vi "test_SessionInitializeErrors_CallCreateSessions_CloseCalledForPreviouslyInitializedSessionsWithProperBehavior.vi"(8 "error in":errorcluster) -> (0 "error out":errorcluster, 2 "result":string, 3 "pass":bool)   [LabVIEW 2020, in "MeasurementServerTests.lvlib"]
uses:
  MeasurementServerTests.lvlib
  da6ffb6f-c1c9-4957-84dd-e9228483c454.vi
  ffc64c76-1568-41a3-8328-b9126ac9a28d.vi
  Helpers/Fake Instrument/Fake Instrument.lvclass
  \\tsclient\C/dev/measurementlink-labview/Source/Runtime/MeasurementLink Instrument/IInstrument/IInstrument.lvclass
  Runtime/MeasurementLink Session Management/Session Reservation/Create Sessions Impl.vi
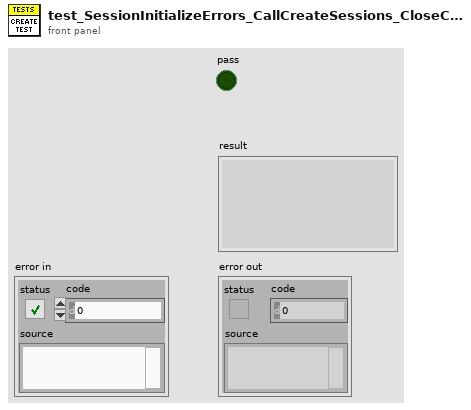
[diagram p1: front panel]
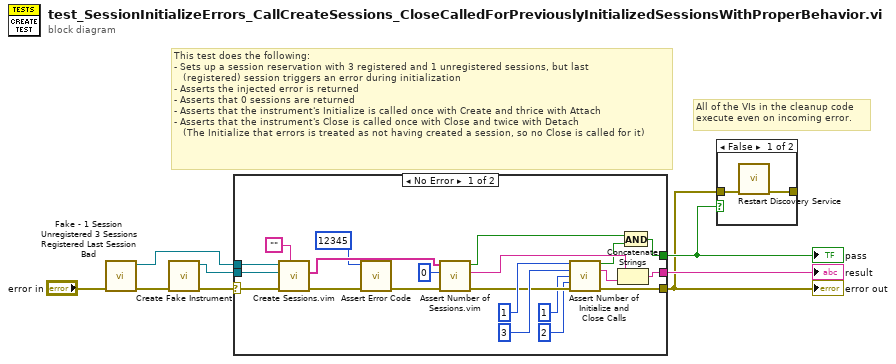
[diagram p0: block diagram]
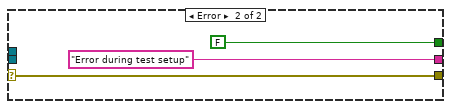
[diagram p2: hidden frame]
diagram:
  # "All of the VIs in the cleanup code\nexecute even on incoming error."
  # "This test does the following:\n- Sets up a session reservation with 3 registered and 1 unregistered sessions, but last\n   (registered) session triggers an error during initialization\n- Asserts the injected error is returned\n- Asserts that 0 sessions are returned\n- Asserts that the instrument's Initialize is called once with Create and thrice with Attach\n- Asserts that the instrument's Close is called once with Close and twice with Detach\n   (The Initialize that errors is treated as not having created a session, so no Close is called for it)"
  n1 = call "Fake - 1 Session Unregistered 3 Sessions Registered Last Session Bad.vi"("error in"="error in") -> ("error out"=w2:errorcluster, "session reservation out"=w1:refnum<class "Session Reservation.lvclass">)  [unwired: 9 in]
  n2 = call "Create Fake Instrument.vi"("error in"=w2) -> ("error out"=w5:errorcluster, "fake instrument out"=w4:refnum<class "Fake Instrument.lvclass">)  [unwired: 9 in]
  n3 = case shown="No Error" w5 {
    selector: w5 -> [w27 w30]
    tunnel: [w17 w30] -> w6
    tunnel: [w16 FALSE] -> w7
    tunnel: [w14 "Error during test setup" ("f")] -> w8
    tunnel: w4 -> [w29 _]
    tunnel: w1 -> [w28 _]
    frame No Error {
      n4 = call "Create Sessions.vim"("session type"="", "error in"=w27, "instrument"=w29, "session reservation in"=w28) -> ("error out"=w26:errorcluster, "sessions"=w24:string[])  [unwired: 4 in, 2 out]
      n5 = call "Assert Error Code.vi"("error in"=w26, "expected error code"=12345) -> ("error out"=w10:errorcluster)  [unwired: 7 in, 2 out]
      n6 = call "Assert Number of Sessions.vim"("error in"=w10, "expected number of sessions"=0, "sessions"=w24) -> ("error out"=w18:errorcluster, "result"=w23:string, "pass"=w22:bool)  [unwired: 6 in]
      n7 = call "Assert Number of Initialize and Close Calls.vi"("expected initialize-create calls"=u32 1, "expected initialize-attach calls"=u32 3, "expected close-close calls"=u32 1, "expected close-detach calls"=u32 2, "error in"=w18) -> ("pass"=w15:bool, "result"=w13:string, "error out"=w17:errorcluster)  [unwired: 8 in]
      n8 = Concatenate Strings(w23, w13) -> (w14:string)
      n9 = And(x=w22, y=w15) -> (x .and. y?=w16:bool)
    }
    frame Error {
    }
  }
  "error out" <- w6
  "pass" <- w7
  "result" <- w8
  n10 = case shown="False" w7 {
    tunnel: w6 -> [w34 _]
    tunnel: [w33 _] -> _
    frame False {
      n11 = call "Restart Discovery Service.vi"("error in"=w34) -> ("error out"=w33:errorcluster)  [unwired: 10 in]
    }
    frame True {
    }
  }
